vi "Matlab_LoadSequence.vi"(11 "Cluster":T1={"Volt"=10.0, "frequency probe"=6.0, "Nhemicycles"=8.0, "X0"=0.0, "Foc"=20.0, "Length"=10.0, "NTrig"=10.0, "Prof"=30.0} {"Prof" format="%#_13g"; "NTrig" format="%#_13g"; "Length" format="%#_13g"; "Foc" format="%#_13g"; "X0" format="%#_13g"; "Nhemicycles" format="%#_13g"; "frequency probe" format="%#_13g"; "Volt" format="%#_13g"}) -> (0 "c":dbl)   [LabVIEW 2015]
panel:
  out "error out":errorcluster
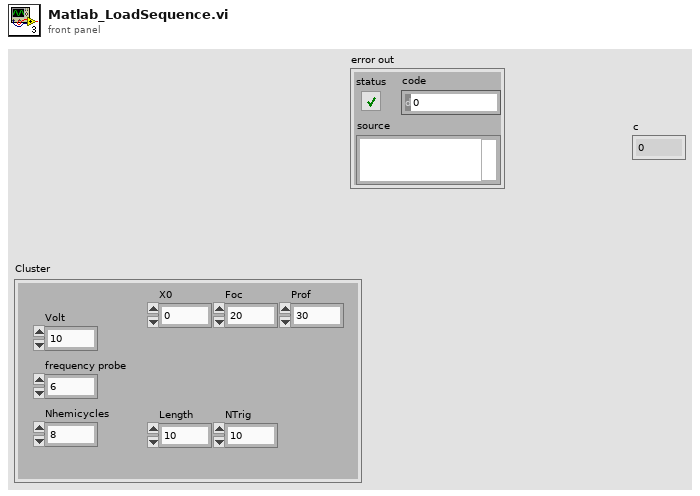
[diagram p1: front panel]
types:
  T1 = cluster{"Volt":dbl, "frequency probe":dbl, "Nhemicycles":dbl, "X0":dbl, "Foc":dbl, "Length":dbl, "NTrig":dbl, "Prof":dbl}
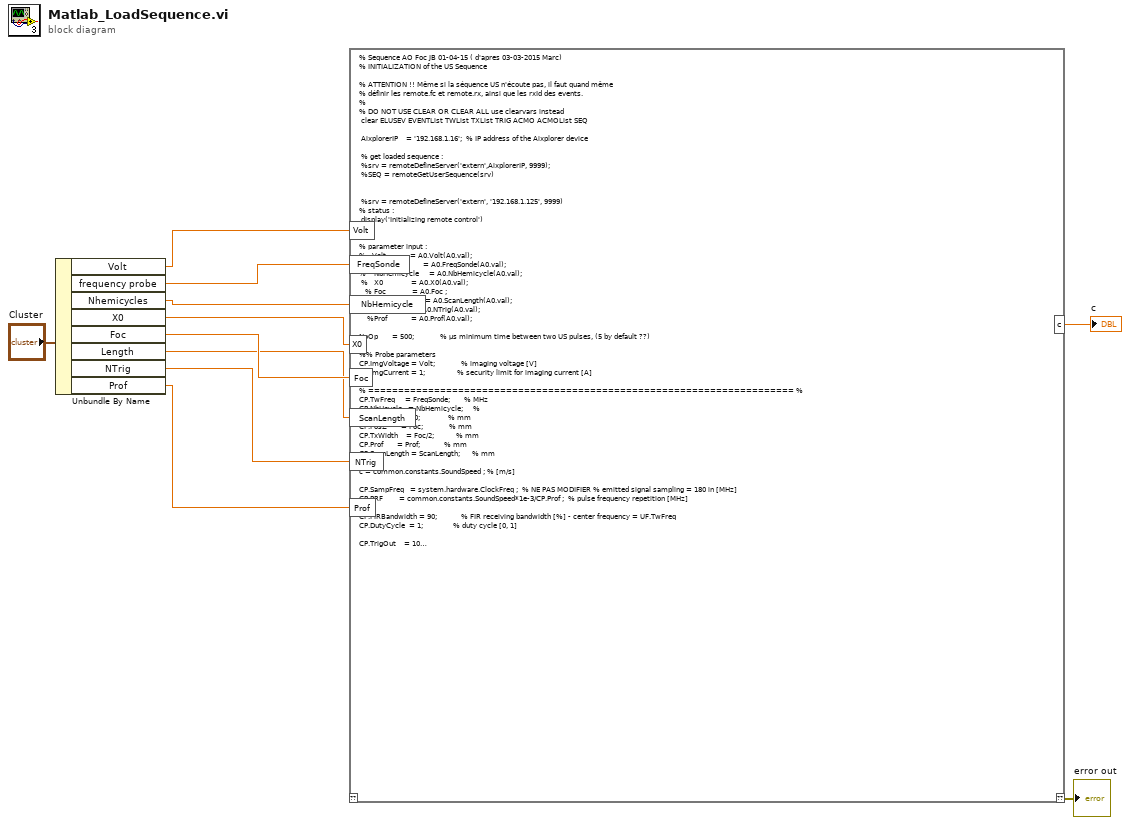
[diagram p0: block diagram]
diagram:
  n1 = Unbundle By Name("Cluster") -> ("Volt"=w8:dbl, "frequency probe"=w7:dbl, "Nhemicycles"=w6:dbl, "X0"=w5:dbl, "Foc"=w4:dbl, "Length"=w3:dbl, "NTrig"=w2:dbl, "Prof"=w1:dbl)
  n2 = script code="% Sequence AO Foc JB 01-04-15 ( d'apres 03-03-2015 Marc)\n% INITIALIZATION of the US Sequence\n\n% ATTENTION !! Même si la séquence US n'écoute pas, il faut quand même\n% définir les remote.fc et remote.rx, ainsi que les rxId des events.\n%\n% DO NOT USE CLEAR OR CLEAR ALL use clearvars instead\n clear ELUSEV EVENTList TWList TXList TRIG ACMO ACMOList SEQ\n\n AixplorerIP    = '192.168.1.16';  % IP address of the Aixplorer device\n \n % get loaded sequence :\n %srv = remoteDefineServer('extern',AixplorerIP, 9999);\n %SEQ = remoteGetUserSequence(srv)\n \n \n %srv = remoteDefineServer('extern', '192.168.1.125', 9999)\n% status :\n display('Initializing remote control')\n\n\n% parameter input :\n%   Volt            = A0.Volt(A0.val);\n%    FreqSonde       = A0.FreqSonde(A0.val);\n%    NbHemicycle     = A0.NbHemicycle(A0.val);\n %   X0              = A0.X0(A0.val);\n   % Foc             = A0.Foc ;\n%    ScanLength      = A0.ScanLength(A0.val);\n  %  NTrig           = A0.NTrig(A0.val);\n    %Prof            = A0.Prof(A0.val);\n\nNoOp       = 500;             % µs minimum time between two US pulses, (5 by default ??)\n\n%% Probe parameters\nCP.ImgVoltage = Volt;             % imaging voltage [V]\nCP.ImgCurrent = 1;                % security limit for imaging current [A]\n\n% ======================================================================= %\nCP.TwFreq     = FreqSonde;       % MHz\nCP.NbHcycle   = NbHemicycle;     %\nCP.PosX       = X0;              % mm\nCP.PosZ       = Foc;             % mm\nCP.TxWidth    = Foc/2;           % mm\nCP.Prof       = Prof;            % mm\nCP.ScanLength = ScanLength;      % mm\n\nc = common.constants.SoundSpeed ; % [m/s]\n\nCP.SampFreq   = system.hardware.ClockFreq ;  % NE PAS MODIFIER % emitted signal sampling = 180 in [MHz]\nCP.PRF        = common.constants.SoundSpeed*1e-3/CP.Prof ;  % pulse frequency repetition [MHz]\n\nCP.FIRBandwidth = 90;            % FIR receiving bandwidth [%] - center frequency = UF.TwFreq\nCP.DutyCycle  = 1;               % duty cycle [0, 1]\n\nCP.TrigOut    = 10; %ceil(CP.Prof/(common.constants.SoundSpeed*1e-3));  %µs ??\nCP.Repeat     = NTrig ;              % a voir\nCP.NoOp       = NoOp ;             % µs minimum time between two US pulses\nCP.Pause      = max(CP.NoOp-ceil(1/CP.PRF),system.hardware.MinNoop); % pause duration in µs\nCP.RxFreq     = 60;              % Receiving center frequency MHz , ??\n\n% ======================================================================= %\n%% Codage en arbitrary : delay matrix and waveform\n\n%actuator pitch :\npitch = system.probe.Pitch ; % in mm\ndt_s = 1/(CP.SampFreq);      % unit us\n\n% Delay [us]\n% c[m/s] -> [mm/us] ; eg factor 1e-3 in the above expression\nDelay = sqrt(CP.PosZ^2+(CP.TxWidth/2)^2)/(c*1e-3) ...\n        - 1/(c*1e-3)*sqrt(CP.PosZ^2+((0:pitch:CP.TxWidth)-CP.TxWidth/2).^2);\n    \n    \n      \n%  figure;\n%  plot(Delay,'r')\n\n% number of steps offset dt_s for each actuators position : \n DlySmpl = round(Delay/dt_s); \n\n % common waveform for emission, square envoppe - non apodized:\n T_Wf = 0:dt_s:0.5*CP.NbHcycle/CP.TwFreq;\n Wf = sin(2*pi*CP.TwFreq*T_Wf); \n \n % number of time-points necessary = points in waveform + maximum delay\n % offset\n N_T = length(Wf) + max(DlySmpl); \n\n%%% construction of a delay matrix : one column / actuator\n WF_mat = zeros(N_T,length(Delay));\n\n for j = 1:length(Delay)\n     % offset for each actuator + normal waveform init\n     WF_mat(DlySmpl(j)+(1:length(Wf)),j) = Wf;\n end\n \n WF_mat_sign = sign(WF_mat); % l'aixplorer code sur 3 niveaux [-1,0,1]\n\n% ======================================================================= %\n%% Arbitrary definition of US events\n% \n% % Elusev\n\n% \n FC = remote.fc('Bandwidth', CP.FIRBandwidth , 0);\n RX = remote.rx('fcId', 1, 'RxFreq', CP.RxFreq, 'QFilter', 2, 'RxElemts', 0, 0);\n\n    if round((CP.PosX+CP.ScanLength)/system.probe.Pitch) > system.probe.NbElemts\n\n        warning('Scan length too long, set to maximum value');\n        CP.ScanLength=system.probe.NbElemts*system.probe.Pitch-CP.PosX;\n\n    end\n\nfor nbs = 1:round(CP.ScanLength/system.probe.Pitch)\n    \n    PosX     = CP.PosX + (nbs-1)*system.probe.Pitch; % center position for the line\n    EvtDur   = ceil(0.5*CP.NbHcycle/CP.TwFreq + max(Delay) + 1/CP.PRF);\n\n    MedElmt  = round(PosX/system.probe.Pitch);\n    \n    TxElemts = MedElmt-round(CP.TxWidth/(2*system.probe.Pitch)):...\n        MedElmt+floor(CP.TxWidth/(2*system.probe.Pitch));\n    \n    WFtmp    = WF_mat_sign( : , ( TxElemts>0 & TxElemts<=system.probe.NbElemts ) );\n    \n    %     figure(471)\n    %     imagesc(WFtmp)\n    %     drawnow\n    \n    % Flat TX\n    TXList{nbs} = remote.tx_arbitrary('txClock180MHz', 1,'twId',nbs,'Delays',0);\n    \n    % Arbitrary TW\n    TWList{nbs} = remote.tw_arbitrary( ...\n        'Waveform',WFtmp', ...\n        'RepeatCH', 0, ...\n        'repeat',0 , ...\n        'repeat256', 0, ...\n        'ApodFct', 'none', ...\n        'TxElemts',TxElemts( TxElemts>0 & TxElemts<=system.probe.NbElemts ), ...\n        'DutyCycle', CP.DutyCycle, ...\n        0);\n    \n    \n    % Event\n    EVENTList{nbs} = remote.event( ...\n        'txId', nbs, ...\n        'rxId', 1, ...\n        'noop', CP.Pause, ...\n        'numSamples', 128, ...\n        'skipSamples', 0, ... 128, ...\n        'duration', EvtDur, ...\n        0);\n    \nend\n\n% % ======================================================================= %\n% %% ELUSEV and ACMO definition\n% % ======================================================================= %\n\nELUSEV = elusev.elusev( ...\n    'tx',           TXList, ...\n    'tw',           TWList, ...\n    'rx',           RX,...\n    'fc',           FC,...\n    'event',        EVENTList, ...\n    'TrigOut',      CP.TrigOut, ... 0,...\n    'TrigIn',       0,...% trigged sequence \n    'TrigAll',      1, ...% 0: sends output trigger at first emission \n    'TrigOutDelay', 0, ...\n    0);\n\nACMO = acmo.acmo( ...\n    'elusev',           ELUSEV, ...\n    'Ordering',         1, ...\n    'Repeat' ,          1, ...\n    'NbHostBuffer',     1, ...\n    'NbLocalBuffer',    1, ...\n    'ControlPts',       900, ... [900 900],...\n    'RepeatElusev',     1, ...\n    0);\n\n ACMOList{1} = ACMO;\n \n% % ======================================================================= %\n% %% Build sequence\n% % ======================================================================= %\n \n% % Probe Param\nTPC = remote.tpc( ...\n    'imgVoltage', CP.ImgVoltage, ...\n    'imgCurrent', CP.ImgCurrent, ...\n    0);\n% \n% % USSE for the sequence\nSEQ = usse.usse( ...\n    'TPC', TPC, ...\n    'acmo', ACMOList, ...    'Loopidx',1, ...\n    'Repeat', CP.Repeat+1, ...    'Popup',0, ...\n    'DropFrames', 0, ...\n    'Loop', 0, ...\n    'DataFormat', 'FF', ...\n    'Popup', 0, ...\n    0);\n\n display('Building sequence to controllor')\n \n [SEQ NbAcq] = SEQ.buildRemote();\n\n display('Build OK')\n \n%%%    Do NOT CHANGE - Sequence execution \n%%%    Initialize remote on systems\n SEQ = SEQ.initializeRemote('IPaddress',AixplorerIP);\n %SEQ.Server\n %SEQ.InfoStruct.event\n \n% remoteGetUserSequence(SEQ.Server)\n% remoteGetStatus(SEQ.Server)\n\n \n display('Remote OK');\n\n % status :\n display('Loading sequence to Hardware');\nSEQ = SEQ.loadSequence();\nSEQ = SEQ.startSequence();\n display('Load OK');\n \n\ndisp('-------------Ready to use-------------------- ')"("Volt"=w8, "FreqSonde"=w7, "NbHemicycle"=w6, "X0"=w5, "Foc"=w4, "ScanLength"=w3, "NTrig"=w2, "Prof"=w1) -> ("??"=→"error out":errorcluster, "c"=→"c":dbl)  [unwired: 1 in]
